vi "Renishaw-XL80_GetHumidity.vi"(8 "error in (no error)":errorcluster, 11 "Renishaw-XL80_EMU in":refnum<class "Renishaw-XL80_EMU.lvclass">) -> (0 "error out":errorcluster, 1 "pStatus":i32(ring) items=["SENSOR_OK"=0, "SENSOR_BAD_READING"=1, "SENSOR_FAILED"=2, "SENSOR_NOT_CONNECTED"=4], 2 "GetHumidity":dbl, 3 "Renishaw-XL80_EMU out":refnum<class "Renishaw-XL80_EMU.lvclass">)   [LabVIEW 2024, in "Renishaw-XL80_EMU.lvclass"]
doc: "This method gets the latest reading (in %RH) and status from the air humidity sensor.\n\nDefinition\nHRESULTGetHumidity( [out] SENSOR_STATUS_CODES *pStatus, [out, retval] double *pVal);\nParameters\npStatus\nA variable that will be set to one of the SENSOR_STATUS_CODES.\n\npVal\nA variable that will be set to the air humidity reading (in %RH).\n\nComments\nIf the client has not connected to the DX10 then the default value (50 %RH) will be returned and the status will be set to SENSOR_NOT_CONNECTED.\n\nIf the client connected to a DX10 and it subsequently stopped responding, or the EC10 stopped responding then the last values obtained from the EC10 will be returned i.e. the status will not be modified. It is important therefore to monitor both the DX10Status and EC10Status. This is easily done using the _RenishawDX10Events interface.\n\nIf the sensor status is SENSOR_NOT_CONNECTED or SENSOR_BAD_READING, then pVal will be set to the last known valid reading.\n\nThe property will normally return an HRESULT of S_OK. However, it will return E_POINTER if the client supplies a null pointer for either pVal or pStatus.\n\nSee"
uses:
  Renishaw-XL80_EMU.lvclass
  <vilib>/numeric/Random Number (Range) DBL.vi
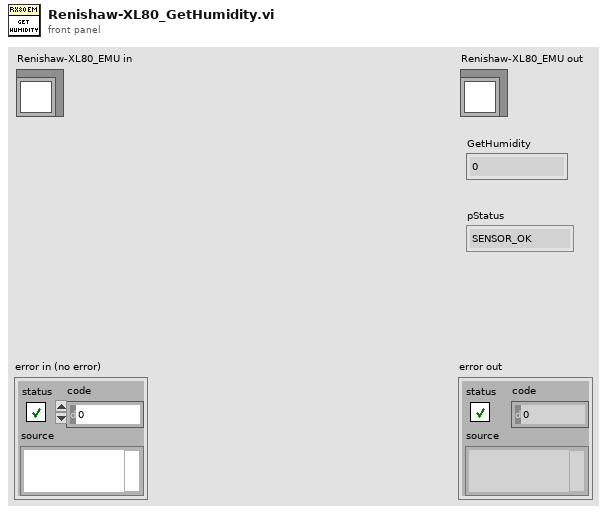
[diagram p1: front panel]
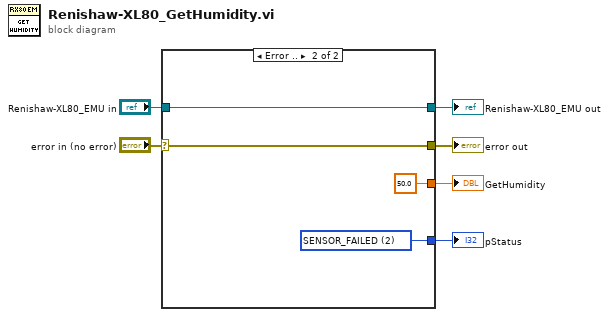
[diagram p0: block diagram]
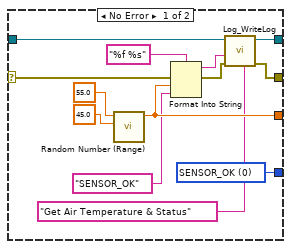
[diagram p2: hidden frame]
diagram:
  n1 = case shown="Error .." "error in (no error)" {
    selector: "error in (no error)" -> [w12 w21]
    tunnel: "Renishaw-XL80_EMU in" -> [w9 w20]
    tunnel: [w17 50.0 ("GetAirTemp")] -> w3
    tunnel: [w16 w22] -> w4
    tunnel: [w8 w21] -> w2
    tunnel: [w7 w20] -> w1
    frame No Error {
      w16 = 0 items=["SENSOR_OK"=0, "SENSOR_BAD_READING"=1, "SENSOR_FAILED"=2, "SENSOR_NOT_CONNECTED"=4] ("pStatus")
      n2 = call-poly <vilib>:"Random Number (Range).vi"("lower bound (0)"=45.0, "upper bound (100)"=55.0) -> ("number"=w17:dbl)  [unwired: 9 in]
      n3 = Format Into String(format string="%f %s", error in=w12, w17, "SENSOR_OK" ("input 2")) -> (resulting string=w14:string, error out=w15:errorcluster)  [unwired: 1 in]
      n4 = call-dynamic "Log_WriteLog.vi"("Additional text"="Get Air Temperature & Status", "error in (no error)"=w15, "Response"=w14, "Log in"=w9) -> ("error out"=w8:errorcluster, "Log out"=w7:refnum<class "Renishaw-XL80_EMU.lvclass">)  [unwired: 6 in]
    }
    frame Error {
      w22 = 2 items=["SENSOR_OK"=0, "SENSOR_BAD_READING"=1, "SENSOR_FAILED"=2, "SENSOR_NOT_CONNECTED"=4] ("pStatus")
    }
  }
  "error out" <- w2
  "Renishaw-XL80_EMU out" <- w1
  "pStatus" <- w4
  "GetHumidity" <- w3
